vi "Get SMO PGSQL Log Paths.vi"(8 "error in (no error)":errorcluster, 11 "Instrument.Oxford1820 in":refnum<class "Instrument.OxfordVRM.lvclass">) -> (0 "error out":errorcluster, 2 "Paths":string, 3 "Instrument.Oxford1820 out":refnum<class "Instrument.OxfordVRM.lvclass">)   [LabVIEW 2016, in "Instrument.OxfordVRM.lvclass"]
uses:
  Instrument.OxfordVRM.lvclass
  Typedefs/getAll.ctl
  <userlib>/LevyLab/Levylab Instruments/Instrument Types/Cryostat/Instrument.Cryostat.lvclass
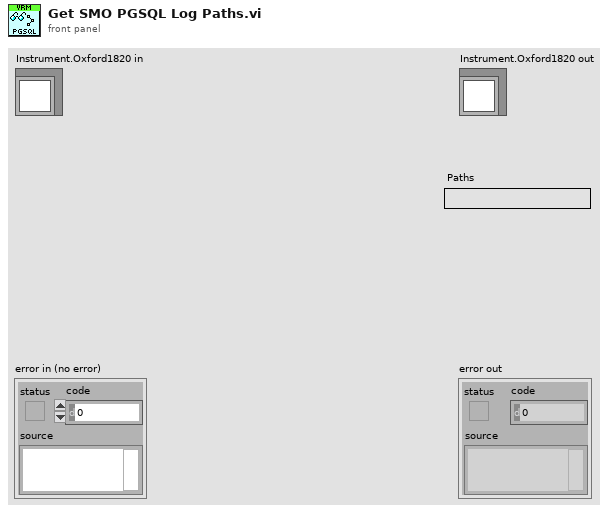
[diagram p1: front panel]
types:
  T1 = typedef "Instrument.OxfordVRM.lvclass/getAll.ctl" = cluster{"Field":dbl[], "Target Field":dbl[], "Target Field Rate":dbl[], "PSU Current":dbl[], "PSU Voltage":dbl[], "Status":string[]}
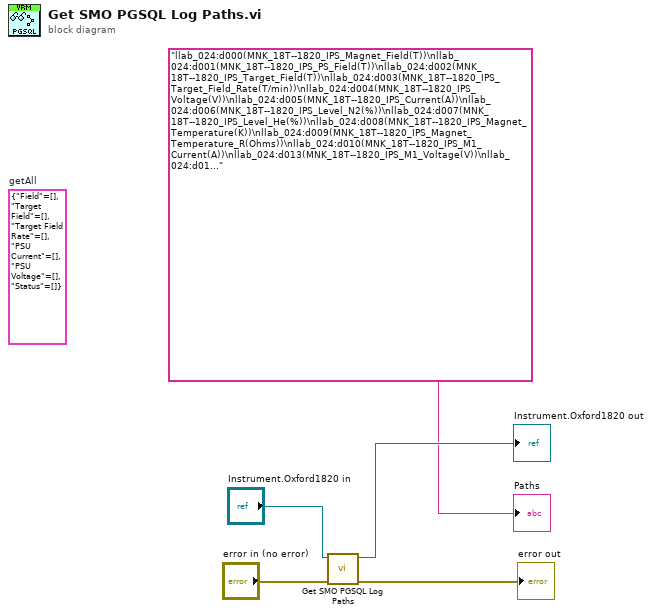
[diagram p0: block diagram]
diagram:
  (unwired) T1 {"Field"=[], "Target Field"=[], "Target Field Rate"=[], "PSU Current"=[], "PSU Voltage"=[], "Status"=[]}  # getAll
  n1 = call-parent "Get SMO PGSQL Log Paths.vi"("error in (no error)"="error in (no error)", "Instrument in"="Instrument.Oxford1820 in") -> ("error out"=→"error out":errorcluster, "Instrument out"=→"Instrument.Oxford1820 out":refnum<class "Instrument.OxfordVRM.lvclass">)  [unwired: 7 in, 1 out]
  "Paths" <- "llab_024:d000(MNK_18T--1820_IPS_Magnet_Field(T))\nllab_024:d001(MNK_18T--1820_IPS_PS_Field(T))\nllab_024:d002(MNK_18T--1820_IPS_Target_Field(T))\nllab_024:d003(MNK_18T--1820_IPS_Target_Field_Rate(T/min))\nllab_024:d004(MNK_18T--1820_IPS_Voltage(V))\nllab_024:d005(MNK_18T--1820_IPS_Current(A))\nllab_024:d006(MNK_18T--1820_IPS_Level_N2(%))\nllab_024:d007(MNK_18T--1820_IPS_Level_He(%))\nllab_024:d008(MNK_18T--1820_IPS_Magnet_Temperature(K))\nllab_024:d009(MNK_18T--1820_IPS_Magnet_Temperature_R(Ohms))\nllab_024:d010(MNK_18T--1820_IPS_M1_Current(A))\nllab_024:d013(MNK_18T--1820_IPS_M1_Voltage(V))\nllab_024:d011(MNK_18T--1820_IPS_M2_Current(A))\nllab_024:d014(MNK_18T--1820_IPS_M2_Voltage(V))\nllab_024:d012(MNK_18T--1820_IPS_M3_Current(A))\nllab_024:d015(MNK_18T--1820_IPS_M3_Voltage(V))\nllab_024:v000(MNK_18T--1820_IPS_Status())\nllab_024:v001(MNK_18T--1820_IPS_Switch())\nllab_024:d016(MNK_18T--1820_ITC_Lambda_Temperature(K))\nllab_024:d017(MNK_18T--1820_ITC_Lambda_Temperature_R(Ohms))\nllab_024:d018(MNK_18T--1820_ITC_Pressure(mbar))\nllab_024:d019(MNK_18T--1820_ITC_Needle_Valve(%))" ("Paths")
